vi "Load From File.vi"(7 "error in (no error)":errorcluster, 9 "File":path, 10 "ByRef Variant Repsitory in":refnum<data-value>) -> (0 "error out":errorcluster)   [LabVIEW 2015, in "ByRef Variant Repository.lvlib"]
uses:
  ByRef Variant Repository.lvlib
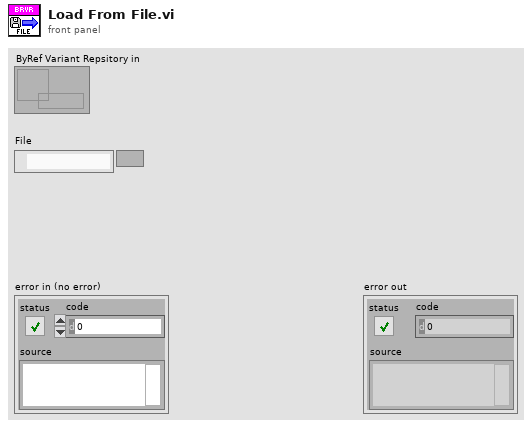
[diagram p1: front panel]
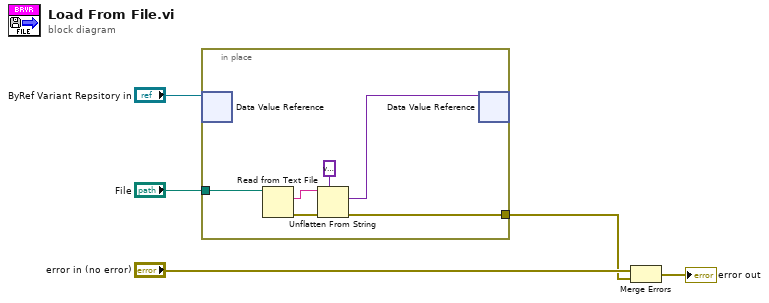
[diagram p0: block diagram]
diagram:
  n1 = in-place {
    in-place-border: "File" -> [w11]
    in-place-border: [w9] -> w1
    n2 = in-place-dvr #1("ByRef Variant Repsitory in") -> ()  [unwired: 2 out]
    n3 = Read from Text File(file (use dialog)=w11) -> (text=w7:string, error out=w10:errorcluster)  [unwired: 3 in, 2 out]
    n4 = Unflatten From String(type=variant, binary string=w7, error in (no error)=w10) -> (value=w6:variant, error out=w9:errorcluster)  [unwired: 2 in, 1 out]
    n5 = in-place-dvr #1(w6) -> ()  [unwired: 2 out]
  }
  n6 = Merge Errors("error in (no error)", w1) -> (→"error out":errorcluster)
